vi "CM-Read Configuration.vi"(0 "Connection File Path":path, 2 "Section":string, 7 "Outputs":string[](array[string]), 11 "error in (no error)":errorcluster) -> (8 "Endpoints":T1[](array[typedef]), 15 "error out":errorcluster)   [LabVIEW 2020]
uses:
  Typedefs/CM-Endpoint.ctl
  <vilib>/Utility/config.llb/Read Key (String).vi
  <vilib>/Utility/config.llb/NI_LVConfig.lvlib
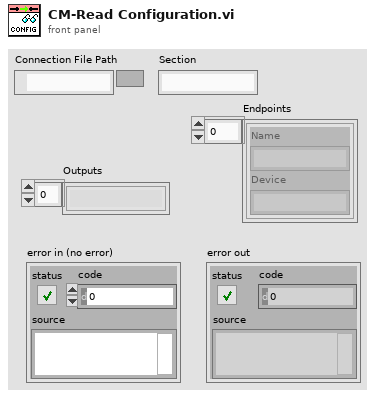
[diagram p1: front panel]
types:
  T1 = typedef "CM-Endpoint.ctl" = cluster{"Name":string, "Device":string}
  T2 = typedef "NI_LVConfig.lvlib/Config Data RefNum.ctl" = refnum<k1>
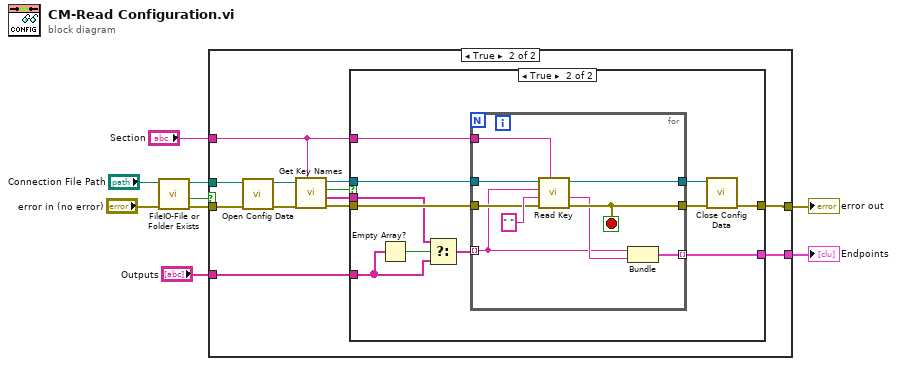
[diagram p0: block diagram]
diagram:
  n1 = call "FileIO-File or Folder Exists.vi"("error in (no error)"="error in (no error)", "path"="Connection File Path") -> ("error out"=w5:errorcluster, "Exists?"=w7:bool, "dup path"=w6:path)  [unwired: 6 in, 1 out]
  n2 = case shown="True" w7 {
    tunnel: w6 -> [_ w22]
    tunnel: w5 -> [w10 w21]
    tunnel: "Section" -> [_ w16]
    tunnel: [w10 w14] -> w3
    tunnel: "Outputs" -> [_ w12]
    tunnel: [_ w13] -> w1
    frame False {
      # "should also be an error"
    }
    frame True {
      n3 = call <vilib>:"Open Config Data.vi"("error in (no error)"=w21, "configuration file path"=w22) -> ("error out"=w19:errorcluster, "refnum"=w20:T2)  [unwired: 7 in, 1 out]
      n4 = call <vilib>:"Get Key Names.vi"("section"=w16, "error in (no error)"=w19, "refnum"=w20) -> ("error out"=w15:errorcluster, "key names"=w17:string[], "section exists?"=w11:bool, "refnum out"=w18:T2)  [unwired: 5 in]
      n5 = case shown="True" w11 {
        tunnel: w18 -> [_ w34]
        tunnel: w17 -> [_ w26]
        tunnel: w16 -> [_ w33]
        tunnel: w15 -> [w23 w32]
        tunnel: [w23 w29] -> w14
        tunnel: [_ w28] -> w13
        tunnel: w12 -> [_ w25]
        frame False {
          # "should be an error"
        }
        frame True {
          n6 = Empty Array?(array=w25) -> (empty?=w27:bool)
          n7 = Select(t=w26, s=w27, f=w25) -> (s? t:f=w24:string[])
          n8 = for {
            tunnel: w34 -> [w43]
            tunnel: [w41] -> w30
            tunnel: w33 -> [w40]
            tunnel: w32 -> [w39]
            tunnel: [w38] -> w31
            tunnel: [w36] -> w28 mode=indexing
            tunnel: w24 -> [w35] mode=indexing
            stop <- w38 stop-if-true
            n9 = call-poly <vilib>:"Read Key.vi"("section"=w40, "error in (no error)"=w39, "default value"=" ", "key"=w35, "refnum"=w43) -> ("error out"=w38:errorcluster, "value"=w37:string, "refnum out"=w41:T2)  [unwired: 3 in, 1 out]
            n10 = Bundle("String"=w35, "value"=w37) -> (w36:cluster{"String":string, "value":string})  [unwired: 1 in]
          }
          n11 = call <vilib>:"Close Config Data.vi"("error in (no error)"=w31, "refnum"=w30) -> ("error out"=w29:errorcluster)  [unwired: 8 in, 1 out]
        }
      }
    }
  }
  "error out" <- w3
  "Endpoints" <- w1
